vi "Calculate Area.vi"(11 "Rectangle":T1) -> (3 "Area":i32)   [LabVIEW 2012]
doc: "Calculates the center of a rectangle"
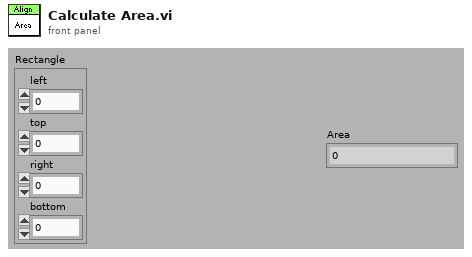
[diagram p1: front panel]
types:
  T1 = cluster{"left":i16, "top":i16, "right":i16, "bottom":i16}
  T2 = cluster{"left":i32, "top":i32, "right":i32, "bottom":i32}
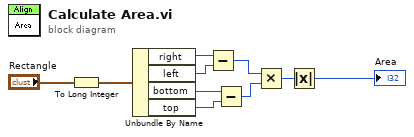
[diagram p0: block diagram]
diagram:
  n1 = To Long Integer(number="Rectangle") -> (32bit integer=w1:T2)
  n2 = Unbundle By Name(w1) -> ("right"=w9:i32, "left"=w8:i32, "bottom"=w7:i32, "top"=w6:i32)
  n3 = Subtract(x=w9, y=w8) -> (x-y=w5:i32)
  n4 = Subtract(x=w7, y=w6) -> (x-y=w4:i32)
  n5 = Multiply(x=w5, y=w4) -> (x*y=w3:i32)
  n6 = Absolute Value(x=w3) -> (abs(x)=→"Area":i32)
